vi "WFS Get Spot Centroids.vi"(8 "error in (no error)":errorcluster {"code" format="%.0x"}, 11 "instrument handle":refnum<visa-resource-name>) -> (0 "error out":errorcluster {"code" format="%.0x"}, 1 "Array Centroid Y":sgl[](array[numeric]) format="%.2p", 2 "Array Centroid X":sgl[](array[numeric]) format="%.2p", 3 "instrument handle out":refnum<visa-resource-name>)   [LabVIEW 2020]
doc: "This VI returns two two-dimensional arrays containing the centroid X and Y positions in pixels calculated by WFS Calc Spots Centr Dia Intens.vi.\n\nNote: WFS Calc Spots Centr Dia Intens.vi is required to run successfully before calculated data can be retrieved."
uses:
  WFS_32.dll
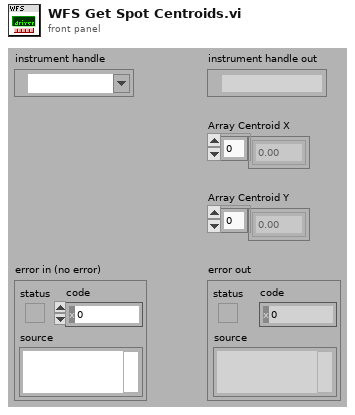
[diagram p1: front panel]
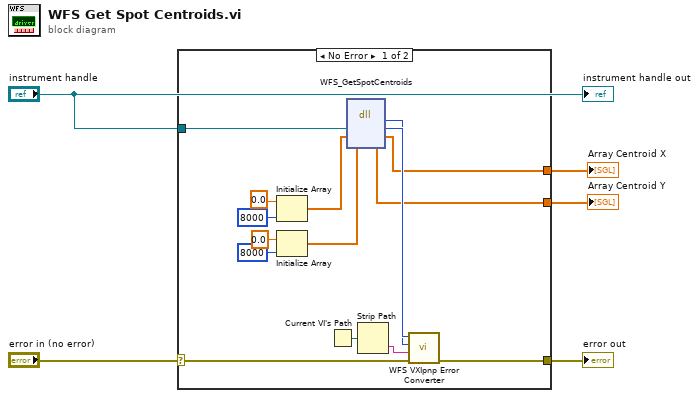
[diagram p0: block diagram]
diagram:
  n1 = case shown="No Error" "error in (no error)" {
    selector: "error in (no error)" -> [w15 w21]
    tunnel: [w14 w21] -> w5
    tunnel: "instrument handle" -> [w19 _]
    tunnel: [w10 _] -> w2
    tunnel: [w6 _] -> w1
    frame No Error {
      n2 = Initialize Array(sgl 0.0 ("element"), 8000 ("dimension size")) -> (w13:sgl[])
      n3 = Initialize Array(sgl 0.0 ("element"), 8000 ("dimension size")) -> (w9:sgl[])
      n4 = Current VI's Path() -> (path=w20:path)
      n5 = dll-call lib="WFS_*.*" fn="WFS_GetSpotCentroids"("Instrument Handle"=w19, "Array Centroid X"=w13, "Array Centroid Y"=w9) -> (w17:i32, "Instrument Handle"=w18:u32, "Array Centroid X"=w10:sgl[], "Array Centroid Y"=w6:sgl[])  [unwired: 3 in, 2 out]
      n6 = Strip Path(path=w20) -> (name=w16:string)  [unwired: 1 out]
      n7 = call "WFS VXIpnp Error Converter.vi"("error in (no error)"=w15, "Name Of VI (\"\")"=w16, "CVI Error Code (0)"=w17, "instrument handle"=w18) -> ("error out"=w14:errorcluster)  [unwired: 6 in, 1 out]
    }
    frame Error {
    }
  }
  "error out" <- w5
  "Array Centroid X" <- w2
  "Array Centroid Y" <- w1
  "instrument handle out" <- "instrument handle"
